vi "Base Error Code.vi"() -> (3 "pximc base error code":i32)   [LabVIEW 2017, in "PXImc.lvlib" / "PXImc Transceiver.lvclass"]
uses:
  PXImc Transceiver.lvclass
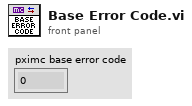
[diagram p1: front panel]
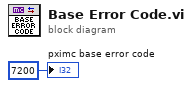
[diagram p0: block diagram]
diagram:
  "pximc base error code" <- 7200 ("pximc base error code")
